vi "temperature_test.vi"() -> ()   [LabVIEW 2019]
panel:
  in  "stop":bool
  out "溫度過低":bool
  out "溫度過高":bool
  out "溫度下限(*C)":dbl
  out "溫度上限(*C)":dbl
  in  "溫度上下限":cluster{dbl, dbl}(slide) scale=0.0..40.0
  out "溫度表":dbl(slide) scale=0.0..40.0
  out "溫度(*C)":dbl format="%#.2g"
  # "溫度計"
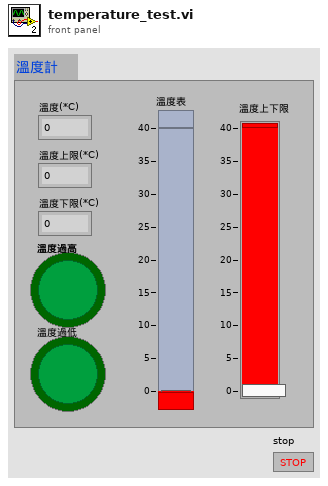
[diagram p1: front panel]
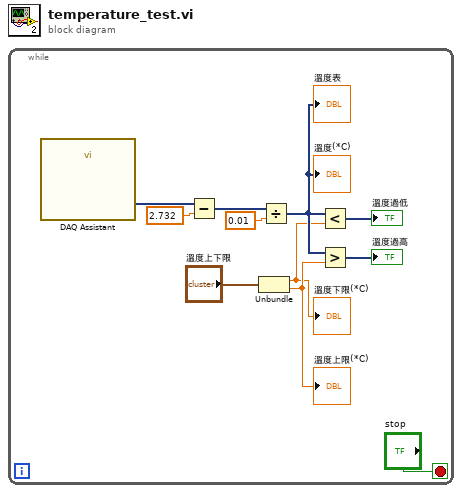
[diagram p0: block diagram]
diagram:
  n1 = while {
    stop <- "stop" stop-if-true
    n2 = call "DAQ Assistant"() -> ("data"=w10:dynamicdata)  [unwired: 17 in, 2 out]
    n3 = Subtract(x=w10, y=2.732) -> (x-y=w8:dynamicdata)
    n4 = Unbundle("溫度上下限") -> (w1:dbl, w2:dbl)
    "溫度上限(*C)" <- w2
    "溫度下限(*C)" <- w1
    n5 = Divide(x=w8, y=0.01) -> (x/y=w5:dynamicdata)
    "溫度(*C)" <- w5
    "溫度表" <- w5
    n6 = Less?(x=w5, y=w1) -> (x < y?=→"溫度過低":dynamicdata)
    n7 = Greater?(x=w5, y=w2) -> (0:→"溫度過高":dynamicdata)
  }
